vi "Text to UTF-8.vi"(8 "error in":errorcluster, 11 "text":string) -> (0 "error out":errorcluster, 3 "utf-8 text":string)   [LabVIEW 2019, in "JSON-RPC.lvclass"]
uses:
  JSON-RPC.lvclass
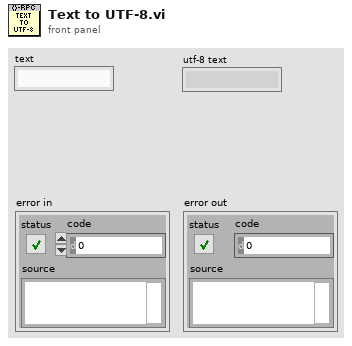
[diagram p1: front panel]
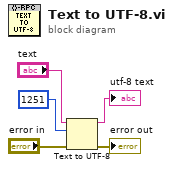
[diagram p0: block diagram]
diagram:
  n1 = Text to UTF-8(8:"error in", 10:1251 ("encoding (system default=-1)"), 11:"text") -> (0:→"error out":errorcluster, 3:→"utf-8 text":string)
